vi "Pre Launch Init Queues.vi"(8 "error in (no error)":errorcluster, 11 "AMS Gas in":refnum<class "AMS Gas.lvclass">) -> (0 "error out":errorcluster, 3 "AMS Gas out":refnum<class "AMS Gas.lvclass">)   [LabVIEW 2015, in "AMS UI.lvlib" / "AMS Gas.lvclass"]
uses:
  AMS Gas.lvclass
  subs/Sample/Sample.lvclass
  AMS Gas.lvclass/AMS Gas.ctl
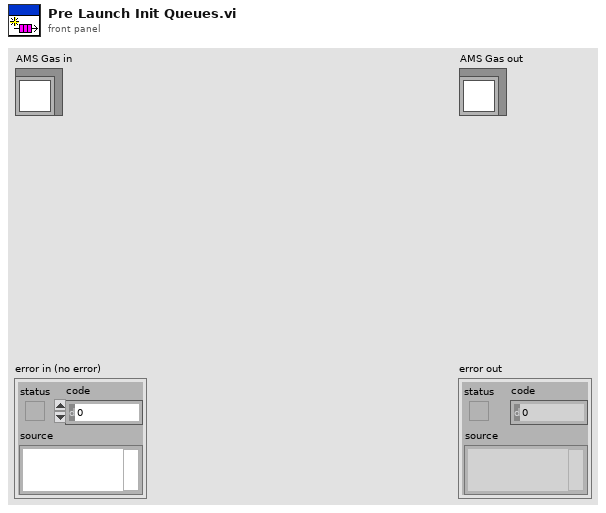
[diagram p1: front panel]
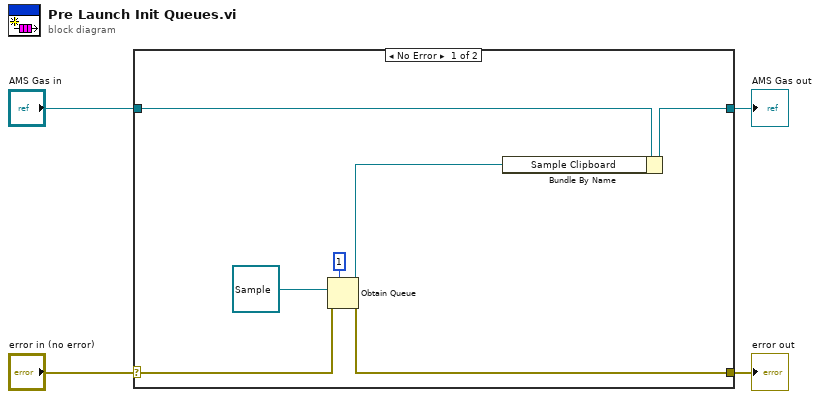
[diagram p0: block diagram]
diagram:
  n1 = case shown="No Error" "error in (no error)" {
    selector: "error in (no error)" -> [w9 w13]
    tunnel: [w8 w13] -> w3
    tunnel: [w10 w12] -> w1
    tunnel: "AMS Gas in" -> [w11 w12]
    frame No Error {
      n2 = Obtain Queue(max queue size (-1, unlimited)=1, element data type=refnum<class "Sample.lvclass"> refnum ("Sample.lvclass"), error in (no error)=w9) -> (queue out=w5:refnum<queue>, error out=w8:errorcluster)  [unwired: 2 in, 1 out]
      n3 = Bundle By Name(cluster=w11, "Sample Clipboard"=w5) -> (w10:refnum<class "AMS Gas.lvclass">)
    }
    frame Error {
    }
  }
  "error out" <- w3
  "AMS Gas out" <- w1
